vi "FGV Config File.vi"(6 "Padrão":string[](array[string]), 8 "Error In":errorcluster, 9 "Standard Path":path, 10 "Set/Get":enum16{"Get", "Set"}(ring)) -> (0 "Error Out":errorcluster, 1 "Padrão Out":string[](array[string]), 2 "Template File":path)   [LabVIEW 2015]
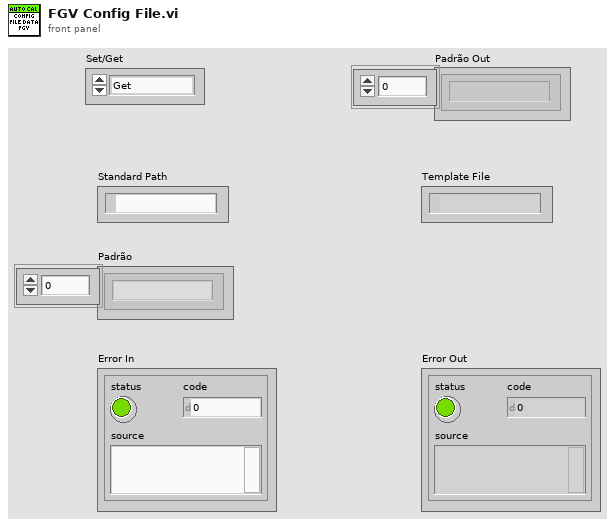
[diagram p1: front panel]
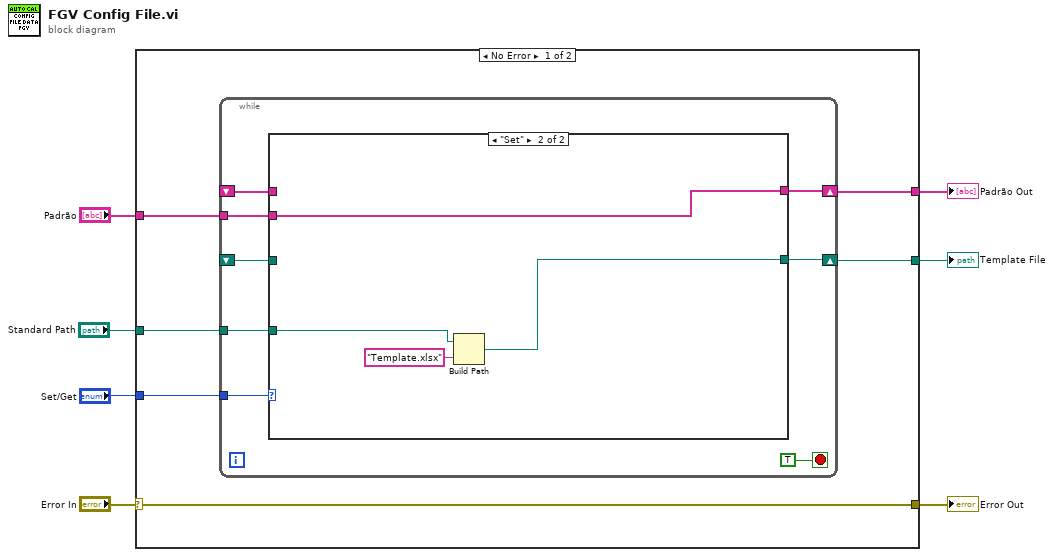
[diagram p0: block diagram]
diagram:
  n1 = case shown="No Error" "Error In" {
    selector: "Error In" -> [w13 w28]
    tunnel: [w13 w28] -> w6
    tunnel: "Set/Get" -> [w12 _]
    tunnel: "Standard Path" -> [w11 _]
    tunnel: [w10 _] -> w3
    tunnel: "Padrão" -> [w9 _]
    tunnel: [w8 _] -> w1
    frame No Error {
      n2 = while {
        tunnel: w12 -> [w20]
        tunnel: w11 -> [w18]
        shift-right: [w19] -> w10
        shift-left: _ -> [w17]
        tunnel: w9 -> [w15]
        shift-right: [w16] -> w8
        shift-left: _ -> [w14]
        stop <- TRUE stop-if-true
        n3 = case shown="\"Set\"" w20 {
          tunnel: [w23 w27] -> w19
          tunnel: w18 -> [_ w24]
          tunnel: w17 -> [w23 _]
          tunnel: [w22 w25] -> w16
          tunnel: w15 -> [_ w25]
          tunnel: w14 -> [w22 _]
          frame "Get", Default {
          }
          frame "Set" {
            n4 = Build Path(base path=w24, name or relative path="Template.xlsx") -> (appended path=w27:path)
          }
        }
      }
    }
    frame Error {
    }
  }
  "Error Out" <- w6
  "Template File" <- w3
  "Padrão Out" <- w1
